vi "close connection.vi"(8 "error in":errorcluster, 11 "TCP master in":refnum<class "IP Data Unit.lvclass">) -> (0 "error out":errorcluster, 3 "TCP master out":refnum<class "IP Data Unit.lvclass">)   [LabVIEW 2021, in "IP Data Unit.lvclass"]
doc: "Closes the TCP connection stored in the class."
uses:
  IP Data Unit.lvclass
  IP Data Unit.lvclass/IP Data Unit.ctl
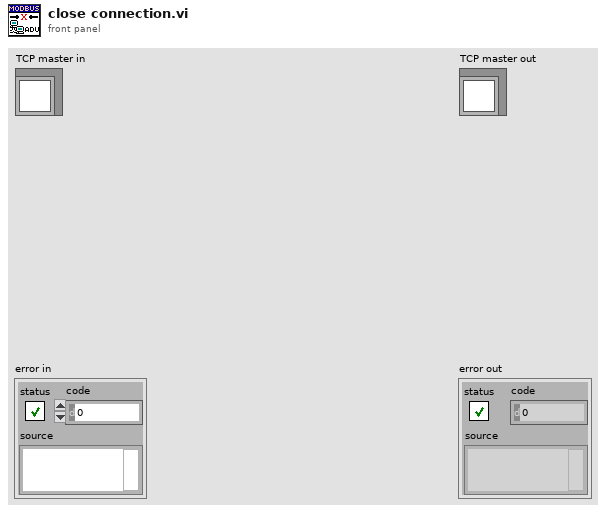
[diagram p1: front panel]
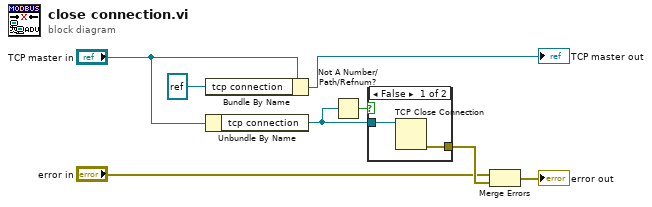
[diagram p0: block diagram]
diagram:
  n1 = Bundle By Name(cluster="TCP master in", "tcp connection"=refnum<k5> refnum) -> (→"TCP master out":refnum<class "IP Data Unit.lvclass">)
  n2 = Unbundle By Name("TCP master in") -> ("tcp connection"=w2:refnum<k5>)
  n3 = Not A Number/Path/Refnum?(number/path/refnum=w2) -> (NaN/Path/Refnum?=w1:bool)
  n4 = case shown="False" w1 {
    tunnel: [w10 _] -> w8
    tunnel: w2 -> [w9 _]
    frame False {
      n5 = TCP Close Connection(connection ID=w9) -> (error out=w10:errorcluster)  [unwired: 2 in, 1 out]
    }
    frame True {
    }
  }
  n6 = Merge Errors("error in", w8) -> (→"error out":errorcluster)
